vi "Base comunicacion serial.vi"() -> ()   [LabVIEW 2021]
uses:
  <vilib>/Instr/_visa.llb/VISA Configure Serial Port (Instr).vi
panel:
  out "substring":string
  in  "Stop Button":bool
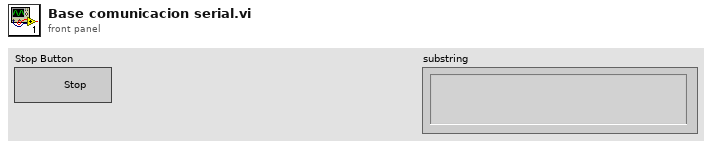
[diagram p1: front panel]
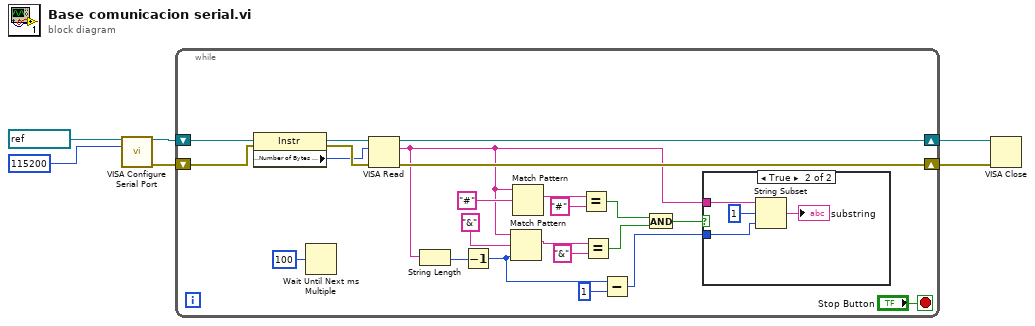
[diagram p0: block diagram]
diagram:
  n1 = call-poly "VISA Configure Serial Port"("VISA resource name"=refnum<visa-resource-name> "COM3", "baud rate (9600)"=u32 115200) -> ("VISA resource name out"=w6:refnum<visa-resource-name>, "error out"=w5:errorcluster)  [unwired: 12 in]
  n2 = while {
    shift-right: [w25] -> w4
    shift-left: w6 -> [w29]
    shift-right: [w24] -> w3
    shift-left: w5 -> [w28]
    stop <- "Stop Button" stop-if-true
    n3 = property class="Instr"(reference=w29, error in=w28) -> (reference out=w27:refnum<visa-resource-name>, error out=w26:errorcluster, "Serial Settings:Number of Bytes at Serial Port"=w23:u32)
    n4 = Wait Until Next ms Multiple(millisecond multiple=u32 100) -> ()  [unwired: 1 out]
    n5 = VISA Read(VISA resource name=w27, byte count=w23, error in (no error)=w26) -> (VISA resource name out=w25:refnum<visa-resource-name>, read buffer=w12:string, error out=w24:errorcluster)  [unwired: 1 out]
    n6 = String Length(string=w12) -> (length=w8:i32)
    n7 = Decrement(x=w8) -> (x-1=w7:i32)
    n8 = Match Pattern(string=w12, regular expression="&", offset (0)=w7) -> (match substring=w16:string)  [unwired: 3 out]
    n9 = Match Pattern(string=w12, regular expression="#") -> (match substring=w19:string)  [unwired: 1 in, 3 out]
    n10 = Equal?(x=w19, y="#") -> (x = y?=w15:bool)
    n11 = Equal?(x=w16, y="&") -> (x = y?=w14:bool)
    n12 = Subtract(x=w7, y=1) -> (x-y=w10:i32)
    n13 = And(x=w15, y=w14) -> (x .and. y?=w13:bool)
    n14 = case shown="True" w13 {
      tunnel: w12 -> [_ w33]
      tunnel: w10 -> [_ w31]
      frame False {
      }
      frame True {
        n15 = String Subset(string=w33, offset (0)=1, length (rest)=w31) -> (substring=→"substring":string)
      }
    }
  }
  n16 = VISA Close(VISA resource name=w4, error in (no error)=w3) -> ()  [unwired: 1 out]
